vi "sub_rplidar_1packet angle-distance.vi"(11 "packet":u8[](array[numeric]) format="%02x") -> (1 "xy":cluster{"x":dbl, "y":dbl}, 2 "angle distance":cluster{"angle":dbl, "distance":dbl}, 3 "udate check":cluster{"update":bool, "check":bool})   [LabVIEW 2019]
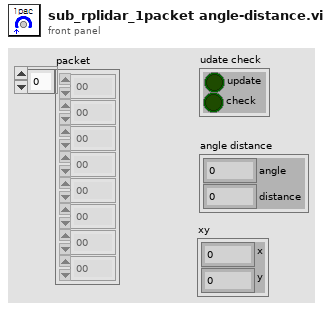
[diagram p1: front panel]
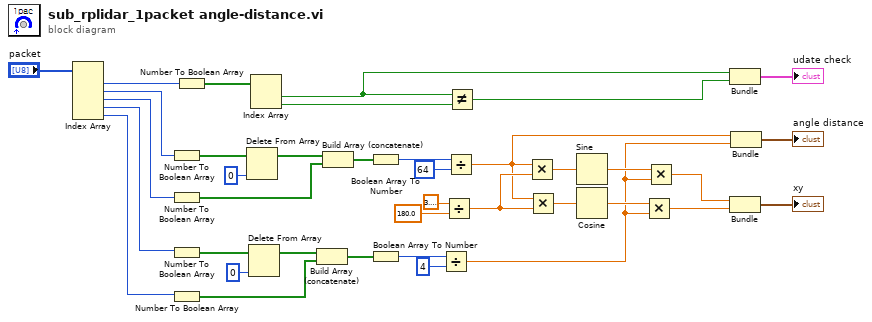
[diagram p0: block diagram]
diagram:
  n1 = Index Array(array="packet") -> (element #1=w24:u8, element #2=w21:u8, element #3=w20:u8, element #4=w19:u8, element #5=w18:u8)  [unwired: 5 in]
  n2 = Number To Boolean Array(number=w21) -> (Boolean array=w38:bool[])
  n3 = Number To Boolean Array(number=w20) -> (Boolean array=w35:bool[])
  n4 = Number To Boolean Array(number=w19) -> (Boolean array=w25:bool[])
  n5 = Number To Boolean Array(number=w18) -> (Boolean array=w28:bool[])
  n6 = Number To Boolean Array(number=w24) -> (Boolean array=w23:bool[])
  n7 = Delete From Array(array=w38, index=0) -> (array with subset deleted=w34:bool[])  [unwired: 1 in, 1 out]
  n8 = Delete From Array(array=w25, index=0) -> (array with subset deleted=w29:bool[])  [unwired: 1 in, 1 out]
  n9 = Index Array(array=w23) -> (element #1=w4:bool, element #2=w22:bool)  [unwired: 2 in]
  n10 = Build Array (concatenate)(w29, w28) -> (w27:bool[])
  n11 = Build Array (concatenate)(w34, w35) -> (w36:bool[])
  n12 = Boolean Array To Number(Boolean array=w36) -> (number=w33:u32)
  n13 = Boolean Array To Number(Boolean array=w27) -> (number=w30:u32)
  n14 = Divide(x=w30, y=u32 4) -> (x/y=w5:dbl)
  n15 = Divide(x=3.141592653589793, y=180.0) -> (x/y=w12:dbl)
  n16 = Divide(x=w33, y=u32 64) -> (x/y=w6:dbl)
  n17 = Not Equal?(x=w4, y=w22) -> (x != y?=w3:bool)
  n18 = Multiply(x=w6, y=w12) -> (x*y=w14:dbl)
  n19 = Multiply(x=w6, y=w12) -> (x*y=w13:dbl)
  n20 = Sine(x=w14) -> (sin(x)=w10:dbl)
  n21 = Cosine(x=w13) -> (cos(x)=w7:dbl)
  n22 = Multiply(x=w7, y=w5) -> (x*y=w8:dbl)
  n23 = Multiply(x=w10, y=w5) -> (x*y=w9:dbl)
  n24 = Bundle(w4, w3) -> (→"udate check":cluster{bool, bool})  [unwired: 1 in]
  n25 = Bundle(w9, w8) -> (→"xy":cluster{dbl, dbl})  [unwired: 1 in]
  n26 = Bundle(w6, w5) -> (→"angle distance":cluster{dbl, dbl})  [unwired: 1 in]
